vi "From JSON Tree.vi"(8 "error in (no error)":errorcluster, 10 "JSON Tree In":variant, 11 "params in":refnum<class "params.lvclass">) -> (0 "error out":errorcluster, 3 "params out":refnum<class "params.lvclass">)   [LabVIEW 2016, in "params.lvclass"]
uses:
  params.lvclass
  params.lvclass/params.ctl
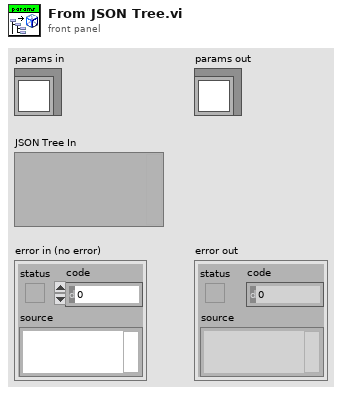
[diagram p1: front panel]
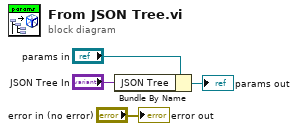
[diagram p0: block diagram]
diagram:
  n1 = Bundle By Name(cluster="params in", "JSON Tree"="JSON Tree In") -> (→"params out":refnum<class "params.lvclass">)
  "error out" <- "error in (no error)"
